vi "write_fifo_resonance.vi"(5 "enable fly-back reversion?":bool, 6 "invert channels":bool[](array[boolean])=[FALSE, FALSE], 7 "fly-back?":bool, 8 "pixel finished?":bool, 10 "maximum bit depth":i8, 11 "integration cluster in":T1) -> (0 "FIFO overflow out":bool, 3 "integration cluster out":T1)   [LabVIEW 2010]
uses:
  integration_cluster.ctl
  <vilib>/rvi/DataTransferAndStorage/Container/XNode/niFpgaContainer.xnode
  <vilib>/rvi/DataTransferAndStorage/Container/Common/niFpgaContainerMethod.ctl
  <vilib>/rvi/DataTransferAndStorage/Container/Common/niFpgaTransferTypeControl.ctl
  <vilib>/rvi/Memory/Memory_Emulation/nirvimemoryEmulationManagerCache_GetValue.vi
  <vilib>/rvi/DataTransferAndStorage/Container/Common/niFpgaContainerGetUniqueNameForEmu.vi
  <vilib>/rvi/Memory/Memory_Emulation/nirvimemoryEmulationManagerCache_InsertValue.vi
  <vilib>/Utility/error.llb/Clear Errors.vi
  <vilib>/rvi/Memory/Memory_Emulation/nirvimemoryEmulationManagerCache_SetValue.vi
  <vilib>/rvi/interface/RandomDataEmulation/nirviRandomDataFPGAFIFO.vi
  <vilib>/rvi/interface/RandomDataEmulation/niFpgaRandomDataHandleErrors.vi
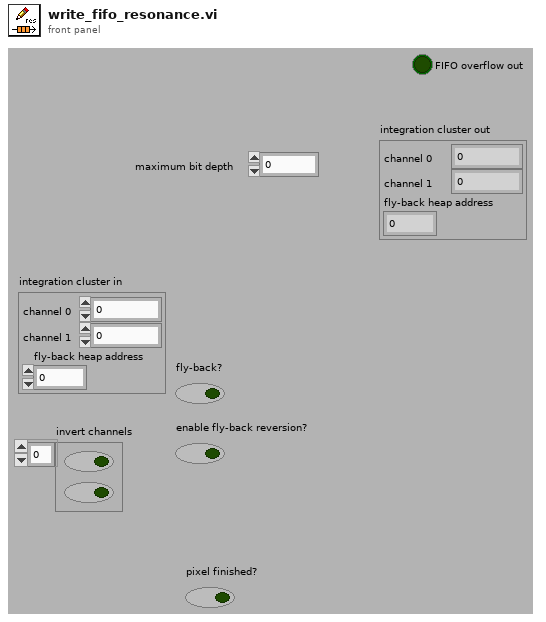
[diagram p1: front panel]
types:
  T1 = typedef "integration_cluster.ctl" = cluster{"channel 0":u32, "channel 1":u32, "fly-back heap address":u32}
  T2 = typedef "niFpgaContainerMethod.ctl" = enum16{"<none>", "write", "read", "clear", "getNumberOfElementsToWrite", "getNumberOfElementsToRead", "enable", "disable", "flushAndDisable", "getStreamState", "readA", "readB", "dramWrite", "dramWriteWithByteEnables", "dramRequestData", "dramRetrieveData"}
  T3 = typedef "niFpgaTransferTypeControl.ctl" = enum16{"Target-Scoped", "Host to Target - DMA", "Target to Host - DMA", "Peer to Peer Reader", "Peer to Peer Writer", "Bidirectional"}
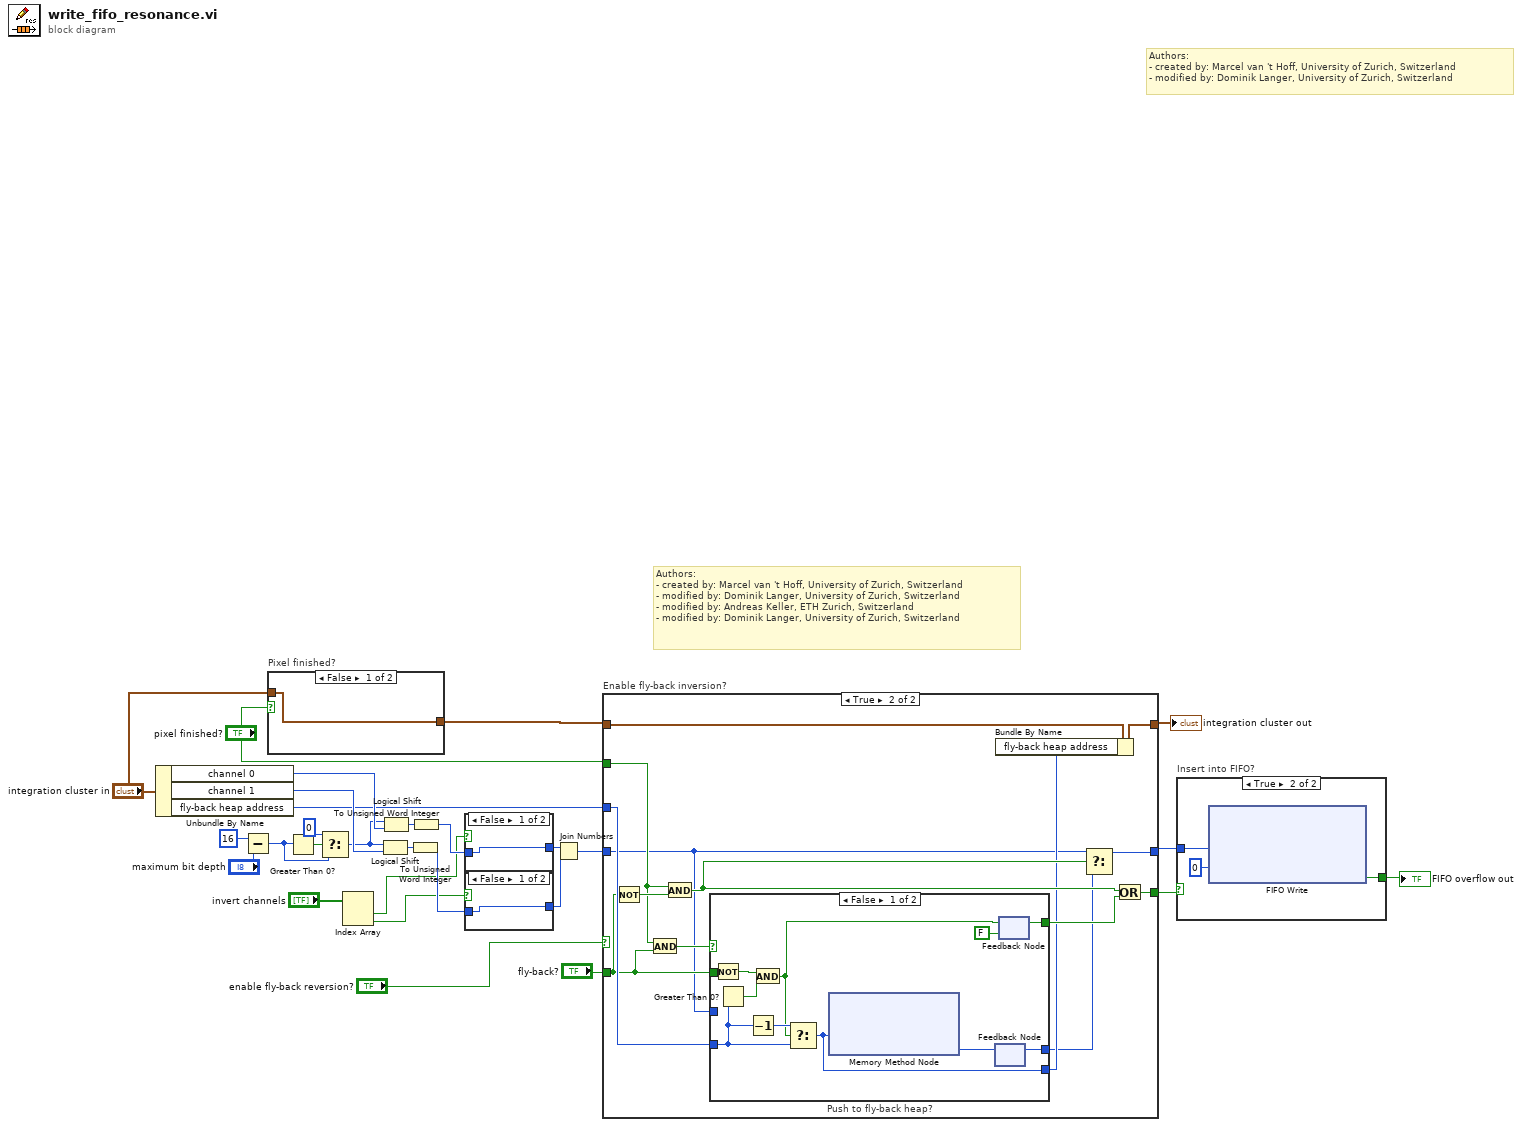
[diagram p0: block diagram]
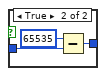
[diagram p2: hidden frame]
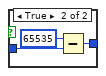
[diagram p3: hidden frame]
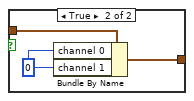
[diagram p4: hidden frame]
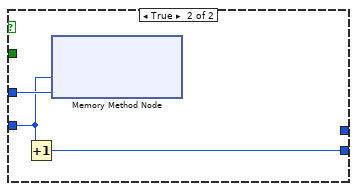
[diagram p6: hidden frame]
diagram:
  # "Authors: \n- created by: Marcel van 't Hoff, University of Zurich, Switzerland\n- modified by: Dominik Langer, University of Zurich, Switzerland\n- modified by: Andreas Keller, ETH Zurich, Switzerland\n- modified by: Dominik Langer, University of Zurich, Switzerland"
  # "Authors: \n- created by: Marcel van 't Hoff, University of Zurich, Switzerland\n- modified by: Dominik Langer, University of Zurich, Switzerland"
  n1 = Unbundle By Name("integration cluster in") -> ("channel 0"=w21:u32, "channel 1"=w22:u32, "fly-back heap address"=w13:u32)
  n2 = Subtract(x=i8 16, y="maximum bit depth") -> (x-y=w24:i8)
  n3 = case "Pixel finished?" shown="False" "pixel finished?" {
    tunnel: "integration cluster in" -> [w29 w31]
    tunnel: [w29 w30] -> w10
    frame False {
    }
    frame True {
      w32 = u32 0 ("channel 1")
      n4 = Bundle By Name(cluster=w31, "channel 0"=w32, "channel 1"=w32) -> (w30:T1)
    }
  }
  n5 = Greater Than 0?(x=w24) -> (x > 0?=w23:bool)
  n6 = Select(t=i8 0 ("f"), s=w23, f=w24) -> (s? t:f=w20:i8)
  n7 = Index Array(array="invert channels") -> (element #1=w2:bool, element #2=w1:bool)  [unwired: 2 in]
  n8 = Logical Shift(y=w20, x=w22) -> (x << y=w19:u32)
  n9 = Logical Shift(y=w20, x=w21) -> (x << y=w18:u32)
  n10 = To Unsigned Word Integer(number=w19) -> (unsigned 16bit integer=w5:u16)
  n11 = To Unsigned Word Integer(number=w18) -> (unsigned 16bit integer=w7:u16)
  n12 = case shown="False" w2 {
    tunnel: [w33 w35] -> w6
    tunnel: w7 -> [w33 w34]
    frame False {
    }
    frame True {
      n13 = Subtract(x=u16 65535, y=w34) -> (x-y=w35:u16)
    }
  }
  n14 = case shown="False" w1 {
    tunnel: [w37 w39] -> w4
    tunnel: w5 -> [w37 w38]
    frame False {
    }
    frame True {
      n15 = Subtract(x=u16 65535, y=w38) -> (x-y=w39:u16)
    }
  }
  n16 = Join Numbers(hi=w6, lo=w4) -> ((hi.lo)=w17:u32)
  n17 = case "Enable fly-back inversion?" shown="True" "enable fly-back reversion?" {
    tunnel: w13 -> [_ w57]
    tunnel: w17 -> [w43 w46]
    tunnel: [w43 w55] -> w16
    tunnel: "pixel finished?" -> [w42 w50]
    tunnel: [w42 w45] -> w12
    tunnel: "fly-back?" -> [_ w52]
    tunnel: w10 -> [w41 w49]
    tunnel: [w41 w47] -> w8
    frame False {
    }
    frame True {
      n18 = Not(x=w52) -> (.not. x?=w56:bool)
      n19 = And(x=w50, y=w52) -> (x .and. y?=w54:bool)
      n20 = And(x=w50, y=w56) -> (x .and. y?=w53:bool)
      n21 = case "Push to fly-back heap?" shown="False" w54 {
        tunnel: w46 -> [_ w197]
        tunnel: [w60 w196] -> w48
        tunnel: w57 -> [w62 w195]
        tunnel: w52 -> [w67 _]
        tunnel: [w64 _] -> w44
        tunnel: [w66 _] -> w51
        frame False {
          n22 = Not(x=w67) -> (.not. x?=w59:bool)
          n23 = Greater Than 0?(x=w62) -> (x > 0?=w68:bool)
          n24 = Decrement(x=w62) -> (x-1=w61:u32)
          n25 = And(x=w59, y=w68) -> (x .and. y?=w58:bool)
          n26 = Select(t=w61, s=w58, f=w62) -> (s? t:f=w60:u32)
          n27 = xnode ("Memory Method Node")("Address"=w60) -> ("Data"=w63:u32)  [unwired: 1 in, 1 out]
          n28 = feedback #1() -> (w64:u32)  [unwired: 1 in]
          n29 = feedback-in #1(w63) -> ()
          n30 = feedback #2(FALSE) -> (w66:bool)
          n31 = feedback-in #2(w58) -> ()
        }
        frame True {
          n32 = Increment(x=w195) -> (x+1=w196:u32)
          n33 = xnode ("Memory Method Node")("Address"=w195, "Data"=w197) -> ()  [unwired: 1 in, 1 out]
        }
      }
      n34 = Bundle By Name(cluster=w49, "fly-back heap address"=w48) -> (w47:T1)
      n35 = Select(t=w46, s=w53, f=w44) -> (s? t:f=w55:u32)
      n36 = Or(x=w53, y=w51) -> (x .or. y?=w45:bool)
    }
  }
  "integration cluster out" <- w8
  n37 = case "Insert into FIFO?" shown="True" w12 {
    tunnel: [_ w325] -> w27
    tunnel: w16 -> [_ w323]
    frame False {
    }
    frame True {
      n38 = xnode ("FIFO Write")("Element"=w323, "Timeout"=0) -> ("Timed Out?"=w325:bool)  [unwired: 1 in, 1 out]
    }
  }
  "FIFO overflow out" <- w27
